vi "CLD 10 Step Sequencer with CSV Solution.vi"() -> ()   [LabVIEW 2020]
doc: "CLD 10 Exercise\n\nUsing the state machine from CLD 9 and the FGV from CLD 6 exercise shortens the development time for this exercise."
uses:
  Controls/CLD 6 CSV file enum.ctl
panel:
  in  "Reset Button":bool
  in  "Auto Reset":bool=TRUE
  in  "Time Target (s)":dbl
  out "Elapsed Time (s)":string
  out "Step 1":bool
  out "Step 3":bool
  out "Step 2":bool
  in  "Stop VI":bool
  out "Current Step Time":dbl
  out "Time Has Elapsed":bool
  out "error out":errorcluster
  in  "error in (no error)":errorcluster
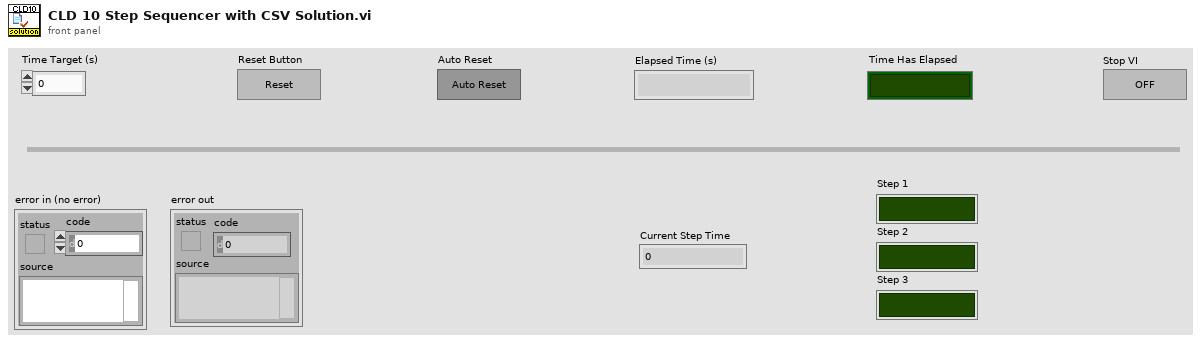
[diagram p1: front panel]
types:
  T1 = typedef "CLD 6 CSV file enum.ctl" = enum16{"Read CSV", "Write CSV"}
  T2 = typedef "CLD 6 CSV file data structure.ctl" = cluster{"Dwell Time":i32, "State 1":bool, "State 2":bool, "State 3":bool}
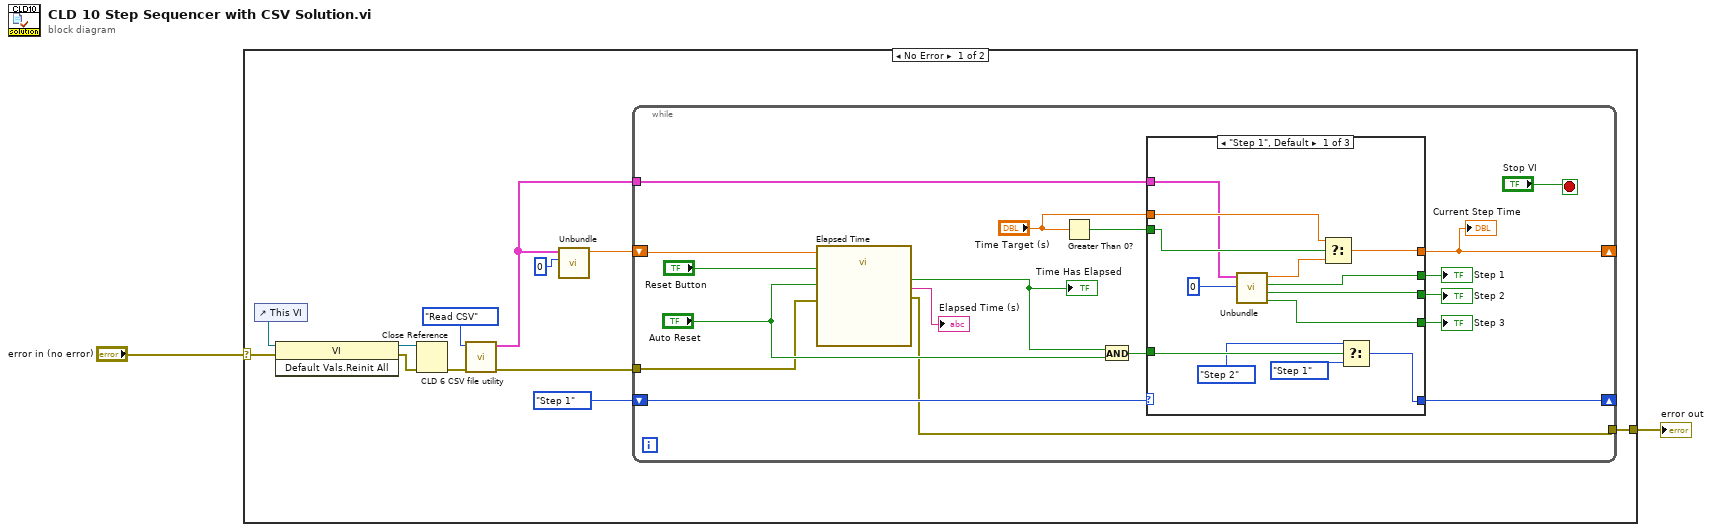
[diagram p0: block diagram]
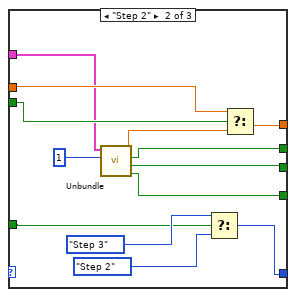
[diagram p2: hidden frame]
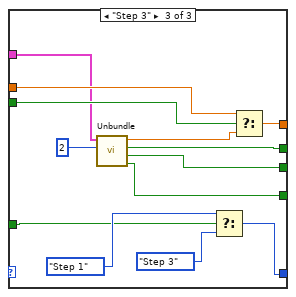
[diagram p3: hidden frame]
diagram:
  n1 = case shown="No Error" "error in (no error)" {
    selector: "error in (no error)" -> [w8 w72]
    tunnel: [w10 w72] -> w1
    frame No Error {
      n2 = control-ref of="This VI"() -> (w12:refnum<vi>)
      n3 = invoke class="VI" method="Default Vals.Reinit All"(reference=w12, error in=w8) -> (reference out=w13:refnum<vi>, error out=w11:errorcluster)  [unwired: 1 in, 1 out]
      n4 = Close Reference(reference=w13, error in (no error)=w11) -> (error out=w5:errorcluster)
      n5 = call "CLD 6 CSV file utility.vi"("Error In"=w5, "CLD 6 file Enum"=CLD_6_CSV_file_enum."Read CSV") -> ("Error Out"=w4:errorcluster, "[Data Out]"=w7:T2[])  [unwired: 8 in]
      n6 = call "Unbundle.vi"("index"=0, "[Data Out]"=w7) -> ("Numeric"=w6:dbl)  [unwired: 6 in, 3 out]
      n7 = while {
        shift-right: [w31] -> _
        shift-left: enum16{"Step 1", "Step 2", "Step 3"}."Step 1" ("f") -> [w32]
        shift-right: [w18] -> _
        shift-left: w6 -> [w30]
        tunnel: [w19] -> w10
        tunnel: w7 -> [w16]
        tunnel: w4 -> [w15]
        stop <- "Stop VI" stop-if-true
        n8 = call "Elapsed Time"("Time Target (s)"=w30, "Reset"="Reset Button", "Auto Reset"="Auto Reset", "error in (no error)"=w15) -> ("Time has Elapsed"=w17:bool, "Elapsed Time Text"=→"Elapsed Time (s)":string, "error out"=w19:errorcluster)  [unwired: 8 in, 5 out]
        "Time Has Elapsed" <- w17
        n9 = Greater Than 0?(x="Time Target (s)") -> (x > 0?=w29:bool)
        n10 = And(x=w17, y="Auto Reset") -> (x .and. y?=w28:bool)
        n11 = case shown="\"Step 1\", Default" w32 {
          tunnel: [w42 w55 w68] -> w31
          tunnel: [w39 w52 w65] -> w18
          tunnel: w28 -> [w45 w56 w69]
          tunnel: w29 -> [w41 w53 w66]
          tunnel: "Time Target (s)" -> [w40 w54 w67]
          tunnel: [w36 w49 w61] -> w23
          tunnel: [w35 w48 w60] -> w22
          tunnel: [w34 w47 w59] -> w21
          tunnel: w16 -> [w38 w51 w64]
          frame "Step 1", Default {
            n12 = call "Unbundle.vi"("index"=0, "[Data Out]"=w38) -> ("State 3"=w34:bool, "State 2"=w35:bool, "State 1"=w36:bool, "Numeric"=w37:dbl)  [unwired: 6 in]
            n13 = Select(t=w40, s=w41, f=w37) -> (s? t:f=w39:dbl)
            n14 = Select(t=enum16{"Step 1", "Step 2", "Step 3"}."Step 2" ("f"), s=w45, f=enum16{"Step 1", "Step 2", "Step 3"}."Step 1") -> (s? t:f=w42:enum16{"Step 1", "Step 2", "Step 3"})
          }
          frame "Step 2" {
            n15 = call "Unbundle.vi"("index"=1, "[Data Out]"=w51) -> ("State 3"=w47:bool, "State 2"=w48:bool, "State 1"=w49:bool, "Numeric"=w46:dbl)  [unwired: 6 in]
            n16 = Select(t=enum16{"Step 1", "Step 2", "Step 3"}."Step 3" ("f"), s=w56, f=enum16{"Step 1", "Step 2", "Step 3"}."Step 2") -> (s? t:f=w55:enum16{"Step 1", "Step 2", "Step 3"})
            n17 = Select(t=w54, s=w53, f=w46) -> (s? t:f=w52:dbl)
          }
          frame "Step 3" {
            n18 = call "Unbundle.vi"("index"=2, "[Data Out]"=w64) -> ("State 3"=w59:bool, "State 2"=w60:bool, "State 1"=w61:bool, "Numeric"=w62:dbl)  [unwired: 6 in]
            n19 = Select(t=enum16{"Step 1", "Step 2", "Step 3"}."Step 1" ("f"), s=w69, f=enum16{"Step 1", "Step 2", "Step 3"}."Step 3") -> (s? t:f=w68:enum16{"Step 1", "Step 2", "Step 3"})
            n20 = Select(t=w67, s=w66, f=w62) -> (s? t:f=w65:dbl)
          }
        }
        "Step 1" <- w23
        "Step 3" <- w21
        "Step 2" <- w22
        "Current Step Time" <- w18
      }
    }
    frame Error {
    }
  }
  "error out" <- w1
